vi "COM Port selector english.vi"() -> (3 "VISA Refnum out":refnum<visa-resource-name>)   [LabVIEW 2020, in "Control de MaP.lvlib"]
uses:
  Control de MaP.lvlib
panel:
  in  "OK Button":bool
  in  "VISA Refnum in":refnum<visa-resource-name>="N/A"
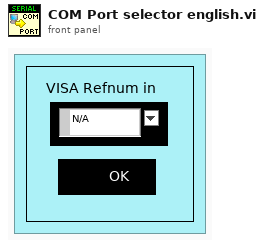
[diagram p1: front panel]
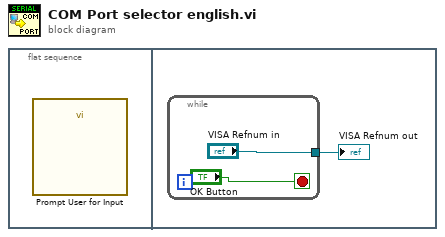
[diagram p0: block diagram]
diagram:
  n1 = flat-sequence {
    frame #0 {
      n2 = call "Prompt User for Input"() -> ()  [unwired: 18 in, 2 out]
    }
    frame #1 {
      n3 = while {
        tunnel: ["VISA Refnum in"] -> w1
        stop <- "OK Button" stop-if-true
      }
      "VISA Refnum out" <- w1
    }
  }
